vi "12-check_version_test.vi"() -> ()   [LabVIEW 2018]
uses:
  LV2Julia_core/VIs/Server or client state.ctl
  LV2Julia_core/VIs/detailed error info.ctl
  LV2Julia_core/VIs/StackFrame.ctl
  LV2Julia_core/VIs/VersionNumber.ctl
  LV2Julia_core/VIs/Commands.ctl
  a521f879-d34e-4576-958d-ff4dfcea3e86.vi
  be4745b6-8471-45fc-b8a0-8968ce92ea4b.vi
  5a89c37d-8165-4bab-9232-2165bf484997.vi
  <vilib>/Utility/High Resolution Relative Seconds.vi
  be4745b6-8471-45fc-b8a0-8968ce92ea4b.vi/01ce1741-ea78-47f8-98ed-e79163fb1a9b.vi
  be4745b6-8471-45fc-b8a0-8968ce92ea4b.vi/01ce1741-ea78-47f8-98ed-e79163fb1a9b.vi/cc3cf2af-bc3b-4fb6-855b-7562c4d0bfeb.vi
  be4745b6-8471-45fc-b8a0-8968ce92ea4b.vi/01ce1741-ea78-47f8-98ed-e79163fb1a9b.vi/c77cecd8-10de-4d46-bc1c-57302a887fda.vi
  be4745b6-8471-45fc-b8a0-8968ce92ea4b.vi/01ce1741-ea78-47f8-98ed-e79163fb1a9b.vi/2cafb1dd-d397-4b79-911a-06d102936120.vi
  LV2Julia_core/VIs/jl-scripts path.vi
  LV2Julia_core/VIs/packages versions global.vi
  LV2Julia_core/VIs/check ID validity.vi
  LV2Julia_core/VIs/bindata_descr to JSON.vi
  LV2Julia_core/VIs/check cluster field names.vi
  LV2Julia_core/VIs/concat JSON.vi
  LV2Julia_core/VIs/build request.vi
  LV2Julia_core/VIs/Parse server response.vi
  LV2Julia_core/VIs/log jl exceptions.vi
  LV2Julia_core/LV2Julia_core.lvlib
panel:
  out "versions":T2
  out "value":cluster{"LVServer_v":T1, "all_current":bool}
  in  "LVServer_min":T1
  in  "LVServer_current":T1
  in  "LV_v":T1
  out "call duration (ms)":dbl format="%#.2f"
  in  "next":bool
  out "detailed error info":T3
  out "current error":errorcluster
  out "final error":errorcluster
  out "short err code":u8
  in  "stop":bool
  out "ZMQ timeout":bool
  out "Julia script file path":path
  out "temporary script path":path
  out "Jl Server state":T5
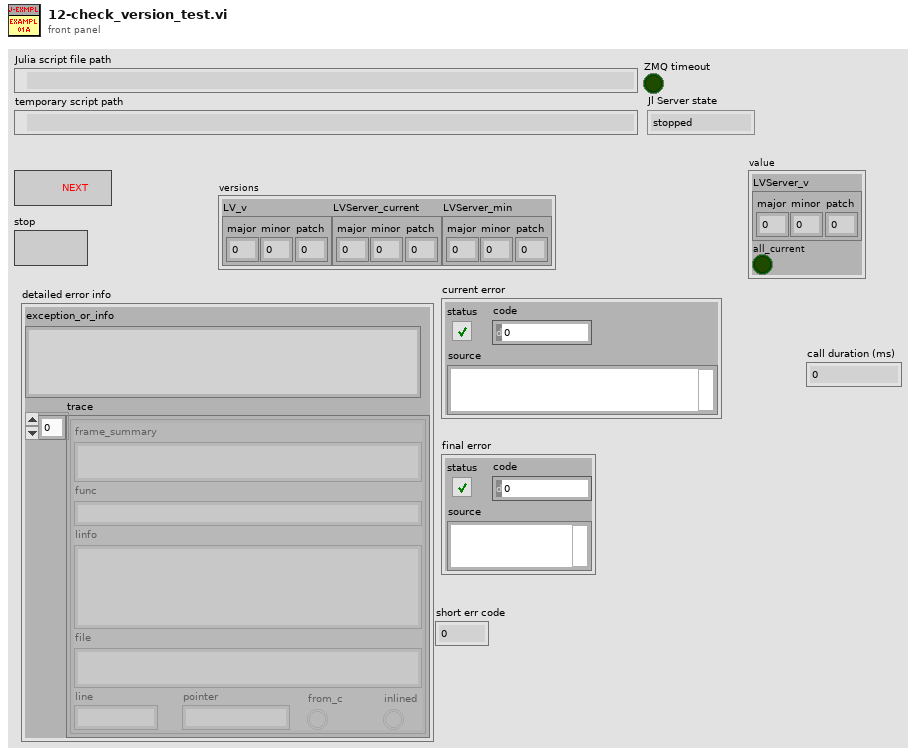
[diagram p1: front panel]
types:
  T1 = typedef "LV2Julia_core.lvlib/VersionNumber.ctl" = cluster{"major":u16, "minor":u16, "patch":u16}
  T2 = cluster{"LV_v":T1, "LVServer_current":T1, "LVServer_min":T1}
  T3 = typedef "LV2Julia_core.lvlib/detailed error info.ctl" = cluster{"exception_or_info":string, "trace":T4[]}
  T4 = typedef "LV2Julia_core.lvlib/StackFrame.ctl" = cluster{"frame_summary":string, "func":string, "linfo":string, "file":string, "line":i32, "pointer":u64, "from_c":bool, "inlined":bool}
  T5 = typedef "LV2Julia_core.lvlib/Server or client state.ctl" = enum16{"stopped", "running", "unknown"}
  T6 = typedef "LV2Julia_core.lvlib/Commands.ctl" = enum16{"Start Jl-server & Init LV-client", "Send request & Get response ", "Stop Jl-server & Cleanup LV-client", "Cleanup LV-client", "Start Jl-server", "Stop Jl-server", "Init LV-Client", "Cleanup LV-Client", "(not allowed)", "Set LV Client state", "Set Jl Server state", "set ZMQ timeout", "read ZMQ timeout", "read-out state"}
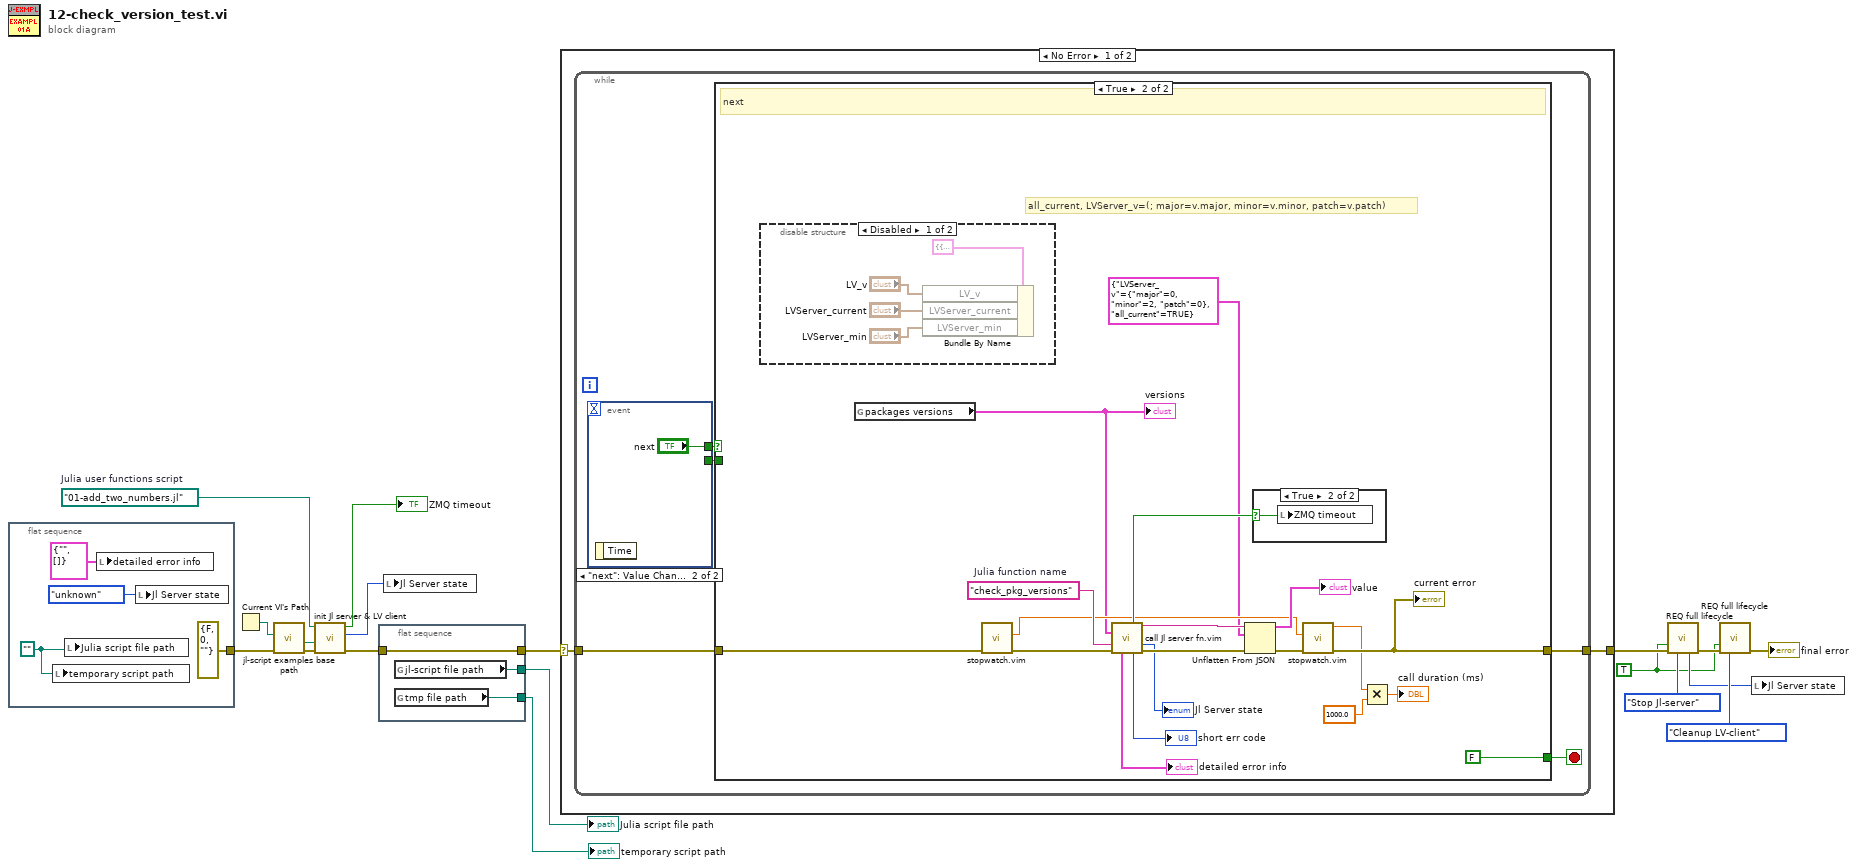
[diagram p0: block diagram]
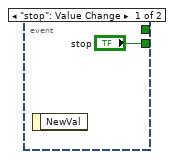
[diagram p2: hidden frame]
diagram:
  w9 = path "01-add_two_numbers.jl"  # Julia user functions script
  w8 = TRUE ("Force command")
  n1 = flat-sequence {
    tunnel: [errorcluster {"status"=FALSE, "code"=0, "source"=""} ("error in (no error)")] -> w4
    frame #0 {
      w19 = path ""
      n2 = local write "temporary script path"(w19) -> ()
      n3 = local write "Julia script file path"(w19) -> ()
      n4 = local write "detailed error info"(T3 {"exception_or_info"="", "trace"=[]} ("detailed error info")) -> ()
      n5 = local write "Jl Server state"(Server_or_client_state."unknown" ("Jl Server state out")) -> ()
    }
  }
  n6 = Current VI's Path() -> (path=w1:path)
  n7 = call "jl-script examples base path.vi"("error in (no error)"=w4, "calling example VI path"=w1) -> ("error out"=w3:errorcluster, "jl-script-examples base path"=w2:path)  [unwired: 8 in]
  n8 = call "init Jl server & LV client.vi"("error in (no error)"=w3, "Base path (not a path)"=w2, "Julia user functions script"=w9) -> ("error out"=w6:errorcluster, "Jl Server state out"=w5:T5, "timeout?"=→"ZMQ timeout":bool)  [unwired: 4 in, 2 out]
  n9 = flat-sequence {
    tunnel: [w25] -> w13
    tunnel: w6 -> [w25]
    tunnel: [w24] -> w11
    tunnel: [w23] -> w12
    frame #0 {
      n10 = global read "jl-scripts path.vi" "jl-script file path"() -> (w24:path)
      n11 = global read "jl-scripts path.vi" "tmp file path"() -> (w23:path)
    }
  }
  n12 = local write "Jl Server state"(w5) -> ()
  n13 = case shown="No Error" w13 {
    selector: w13 -> [w26 w61]
    tunnel: [w27 w61] -> w18
    frame No Error {
      n14 = while {
        tunnel: w26 -> [w31]
        tunnel: [w32] -> w27
        stop <- w29 stop-if-true
        n15 = event shown="[1] \"next\": Value Change" {
          selector: _ -> [_ _]
          dyn-events: _ -> [_ _]
          timeout: _ -> [_ _]
          tunnel: [_ "next"] -> w30
          tunnel: ["stop" _] -> w28
          event "stop": Value Change {
            n16 = event-data() -> ()  [unwired: 1 in, 1 out]
          }
          event "next": Value Change {
            n17 = event-data() -> ()  [unwired: 1 in, 1 out]
          }
        }
        n18 = case shown="True" w30 {
          tunnel: [w36 w41] -> w32
          tunnel: w31 -> [w36 w45]
          tunnel: [w35 FALSE ("stop this VI only")] -> w29
          tunnel: w28 -> [w35 _]
          frame False {
            # "stop"
          }
          frame True {
            w54 = "check_pkg_versions"  # Julia function name
            # "all_current, LVServer_v=(; major=v.major, minor=v.minor, patch=v.patch)"
            # "next"
            n19 = disable-structure shown="Disabled" {
              frame Disabled {
                n20 = Bundle By Name(cluster=T2 {"LV_v"={"major"=0, "minor"=0, "patch"=0}, "LVServer_current"={"major"=0, "minor"=0, "patch"=0}, "LVServer_min"={"major"=0, "minor"=0, "patch"=0}}, "LV_v"="LV_v", "LVServer_current"="LVServer_current", "LVServer_min"="LVServer_min") -> ()  [unwired: 1 out]
              }
              frame Enabled {
              }
            }
            n21 = global read "packages versions global.vi" "packages versions"() -> (w37:T2)
            "versions" <- w37
            n22 = call "stopwatch.vim"("anything in"=w45) -> ("copy of anything out"=w44:errorcluster, "current timepoint"=w40:dbl)  [unwired: 8 in, 1 out]
            n23 = call "call Jl server fn.vim"("Arguments 2"=w37, "fun2call"=w54, "error in (no error)"=w44) -> ("timeout?"=w51:bool, "JSON received"=w48:string, "Jl Server state out"=→"Jl Server state":T5, "detailed error info"=→"detailed error info":T3, "return code"=→"short err code":u8, "error out"=w50:errorcluster)  [unwired: 6 in, 1 out]
            n24 = Unflatten From JSON(JSON string=w48, type and defaults=cluster{"LVServer_v":T1, "all_current":bool} {"LVServer_v"={"major"=0, "minor"=2, "patch"=0}, "all_current"=TRUE}, error in (no error)=w50) -> (value=→"value":cluster{"LVServer_v":T1, "all_current":bool}, error out=w42:errorcluster)  [unwired: 4 in]
            n25 = case shown="True" w51 {
              selector: w51 -> [_ w60]
              frame False {
              }
              frame True {
                n26 = local write "ZMQ timeout"(w60) -> ()
              }
            }
            n27 = call "stopwatch.vim"("anything in"=w42, "prev timepoint (0)"=w40) -> ("copy of anything out"=w41:errorcluster, "delta t (s)"=w39:dbl)  [unwired: 7 in, 1 out]
            "current error" <- w41
            n28 = Multiply(x=w39, y=1000.0) -> (x*y=→"call duration (ms)":dbl)
          }
        }
      }
    }
    frame Error {
    }
  }
  n29 = call "REQ full lifecycle.vi"("Force command"=w8, "error in"=w18, "command"=Commands."Stop Jl-server") -> ("Jl Server state out"=w10:T5, "error out"=w16:errorcluster)  [unwired: 6 in, 5 out]
  n30 = call "REQ full lifecycle.vi"("Force command"=w8, "error in"=w16, "command"=Commands."Cleanup LV-client") -> ("error out"=→"final error":errorcluster)  [unwired: 6 in, 6 out]
  n31 = local write "Jl Server state"(w10) -> ()
  "temporary script path" <- w12
  "Julia script file path" <- w11
